vi "PUMP_change_pressure_slow.vi"(4 "FRP out":T1, 5 "error in":errorcluster, 6 "Pressure setpoint":dbl, 7 "t0":dbl, 8 "MFCS_EZ":T2) -> (0 "error out":errorcluster, 3 "FR Data":cluster{"time (s)":dbl, "volume (µl)":dbl})   [LabVIEW 2015]
uses:
  <userlib>/Fluigent/Fluigent MFCS/FluigentMFCS_Full.llb/_EZmfcsRefNum.ctl
  <userlib>/Fluigent/Fluigent MFCS/FluigentMFCS_Full.llb/_EZmfcsEnum.ctl
  <userlib>/Fluigent/Fluigent FRP/FluigentFRP.llb/_frpEnum.ctl
  <userlib>/Fluigent/Fluigent MFCS/FluigentMFCS_Full.llb/MFCS_EZ Write Channel Pressure.vi
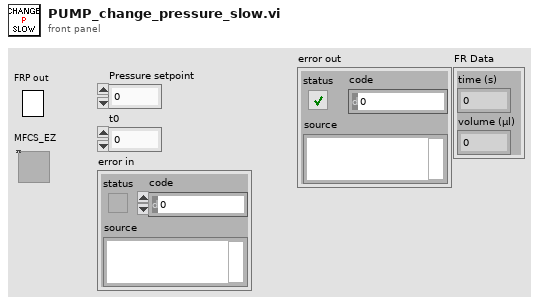
[diagram p1: front panel]
types:
  T1 = typedef "_frpRefNum" = refnum<k1>
  T2 = typedef "_EZmfcsRefNum.ctl" = refnum<k1>
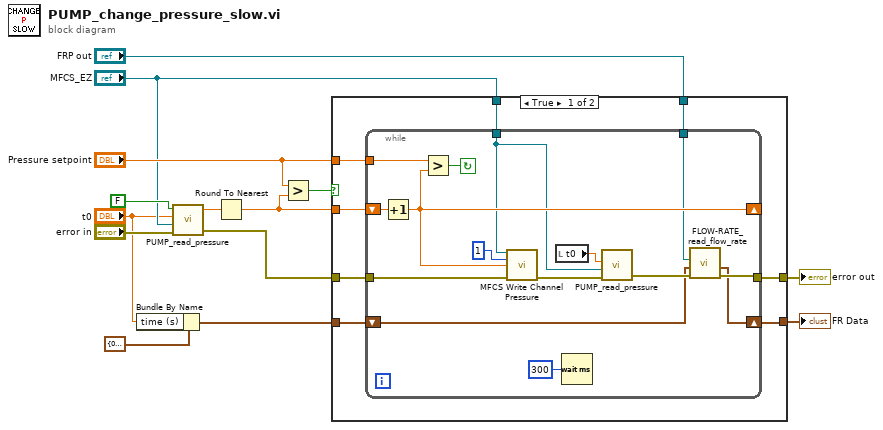
[diagram p0: block diagram]
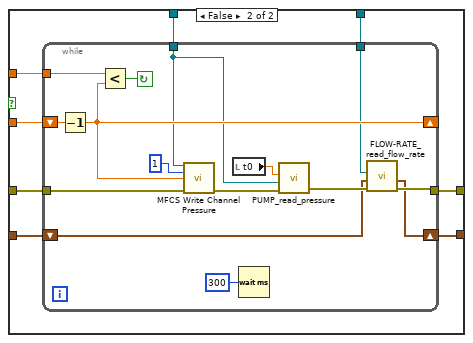
[diagram p2: hidden frame]
diagram:
  n1 = Bundle By Name(cluster=cluster{"time (s)":dbl, "volume (µl)":dbl} {"time (s)"=0.0, "volume (µl)"=0.0} ("Data t i-1"), "time (s)"="t0") -> (w3:cluster{"time (s)":dbl, "volume (µl)":dbl})
  n2 = call "PUMP_read_pressure.vi"("error in"="error in", "MFCS_EZ"="MFCS_EZ", "t0"="t0", "Reset"=FALSE) -> ("error out"=w10:errorcluster, "Pressure (mBar)"=w12:dbl)  [unwired: 1 out]
  n3 = Round To Nearest(number=w12) -> (nearest integer value=w6:dbl)
  n4 = Greater?(x="Pressure setpoint", y=w6) -> (0:w11:bool)
  n5 = case shown="True" w11 {
    tunnel: w10 -> [w20 w43]
    tunnel: w6 -> [w22 w44]
    tunnel: "Pressure setpoint" -> [w21 w45]
    tunnel: [w19 w39] -> w8
    tunnel: "MFCS_EZ" -> [w18 w41]
    tunnel: "FRP out" -> [w17 w40]
    tunnel: w3 -> [w16 w42]
    tunnel: [w15 w38] -> w1
    frame True {
      n6 = while {
        shift-right: [w33] -> _
        shift-left: w22 -> [w37]
        tunnel: w21 -> [w36]
        tunnel: w20 -> [w34]
        tunnel: [w26] -> w19
        tunnel: w18 -> [w28]
        tunnel: w17 -> [w25]
        shift-right: [w23] -> w15
        shift-left: w16 -> [w24]
        stop <- w35 continue-if-true
        n7 = Increment(x=w37) -> (x+1=w33:dbl)
        n8 = Greater?(x=w36, y=w33) -> (0:w35:bool)
        n9 = call-poly <userlib>:"MFCS Write Channel Pressure.vi"("MFCS_EZ"=w28, "Channel Number (default=1)"=u8 1, "Pressure (mBar)"=w33, "error in (no error)"=w34) -> ("error out"=w30:errorcluster)  [unwired: 10 in, 1 out]
        n10 = local read "t0"() -> (w29:dbl)
        n11 = Wait (ms)(milliseconds to wait=u32 300) -> ()  [unwired: 1 out]
        n12 = call "PUMP_read_pressure.vi"("error in"=w30, "MFCS_EZ"=w28, "t0"=w29) -> ("error out"=w27:errorcluster)  [unwired: 1 in, 2 out]
        n13 = call "FLOW-RATE_read_flow_rate.vi"("error in"=w27, "Data t i-1"=w24, "FRP out"=w25) -> ("error out"=w26:errorcluster, "Data t i"=w23:cluster{"time (s)":dbl, "volume (µl)":dbl})  [unwired: 1 in, 2 out]
      }
    }
    frame False {
      n14 = while {
        shift-right: [w56] -> _
        shift-left: w44 -> [w60]
        tunnel: w45 -> [w59]
        tunnel: w43 -> [w57]
        tunnel: [w49] -> w39
        tunnel: w41 -> [w51]
        tunnel: w40 -> [w48]
        shift-right: [w46] -> w38
        shift-left: w42 -> [w47]
        stop <- w58 continue-if-true
        n15 = Decrement(x=w60) -> (x-1=w56:dbl)
        n16 = Less?(x=w59, y=w56) -> (x < y?=w58:bool)
        n17 = call-poly <userlib>:"MFCS Write Channel Pressure.vi"("MFCS_EZ"=w51, "Channel Number (default=1)"=u8 1, "Pressure (mBar)"=w56, "error in (no error)"=w57) -> ("error out"=w53:errorcluster)  [unwired: 10 in, 1 out]
        n18 = local read "t0"() -> (w52:dbl)
        n19 = Wait (ms)(milliseconds to wait=u32 300) -> ()  [unwired: 1 out]
        n20 = call "PUMP_read_pressure.vi"("error in"=w53, "MFCS_EZ"=w51, "t0"=w52) -> ("error out"=w50:errorcluster)  [unwired: 1 in, 2 out]
        n21 = call "FLOW-RATE_read_flow_rate.vi"("error in"=w50, "Data t i-1"=w47, "FRP out"=w48) -> ("error out"=w49:errorcluster, "Data t i"=w46:cluster{"time (s)":dbl, "volume (µl)":dbl})  [unwired: 1 in, 2 out]
      }
    }
  }
  "error out" <- w8
  "FR Data" <- w1
